vi "Copy_File_to_C.vi"(8 "error in (no error)":errorcluster, 9 "Folder":string, 10 "path from":path, 11 "GeneralFunctionality in":refnum<class "GeneralFunctionality.lvclass">) -> (0 "error out":errorcluster, 2 "appended path out":path, 3 "GeneralFunctionality out":refnum<class "GeneralFunctionality.lvclass">)   [LabVIEW 2019, in "GeneralFunctionality.lvclass"]
uses:
  GeneralFunctionality.lvclass
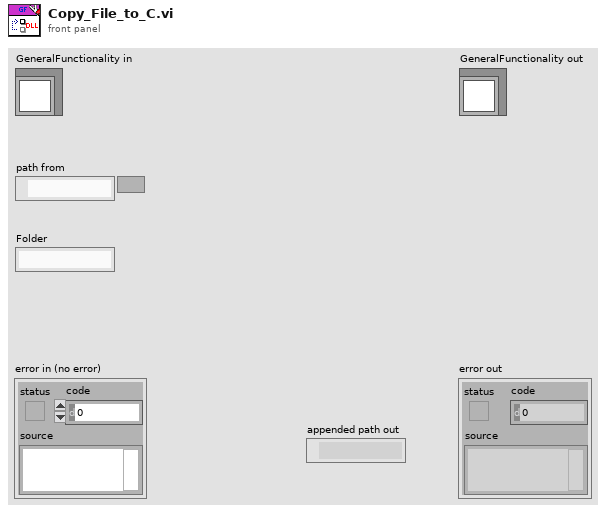
[diagram p1: front panel]
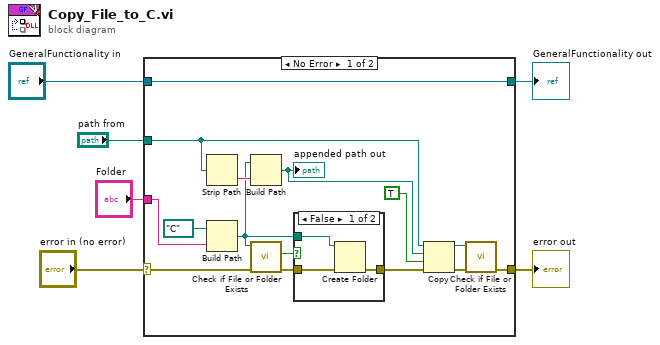
[diagram p0: block diagram]
diagram:
  n1 = case shown="No Error" "error in (no error)" {
    selector: "error in (no error)" -> [w12 w27]
    tunnel: [w11 w27] -> w5
    tunnel: [w21 w26] -> w3
    tunnel: "GeneralFunctionality in" -> [w21 w26]
    tunnel: "Folder" -> [w9 _]
    tunnel: "path from" -> [w7 _]
    frame No Error {
      n2 = Strip Path(path=w7) -> (name=w13:string)  [unwired: 1 out]
      n3 = Build Path(base path=path "C:/" ("appended path"), name or relative path=w9) -> (appended path=w8:path)
      n4 = Build Path(base path=w8, name or relative path=w13) -> (appended path=w20:path)
      "appended path out" <- w20
      n5 = call <vilib>:"Check if File or Folder Exists.vi"("error in (no error)"=w12, "path"=w8) -> ("error out"=w19:errorcluster, "file or folder exists?"=w17:bool)  [unwired: 7 in, 1 out]
      n6 = case shown="False" w17 {
        tunnel: [w22 w25] -> w18
        tunnel: w19 -> [w23 w25]
        tunnel: w8 -> [w24 _]
        frame False {
          n7 = Create Folder(path (use dialog)=w24, error in=w23) -> (error out=w22:errorcluster)  [unwired: 1 in, 2 out]
        }
        frame True {
        }
      }
      n8 = Copy(8:w18, 9:TRUE ("overwrite (F)"), 10:w20, 11:w7) -> (0:w15:errorcluster, 3:w14:path)  [unwired: 1 in, 1 out]
      n9 = call <vilib>:"Check if File or Folder Exists.vi"("error in (no error)"=w15, "path"=w14) -> ("error out"=w11:errorcluster)  [unwired: 7 in, 2 out]
    }
    frame Error {
    }
  }
  "error out" <- w5
  "GeneralFunctionality out" <- w3
